vi "Is TLS.vi"(8 "error in (no error)":errorcluster, 11 "WebsocketStream in":refnum<class "WebsocketStream.lvclass">) -> (0 "error out":errorcluster, 2 "Is TLS?":bool, 3 "WebsocketStream out":refnum<class "WebsocketStream.lvclass">)   [LabVIEW 2020, in "Stream-Websocket.lvlib" / "WebsocketStream.lvclass"]
uses:
  WebsocketStream.lvclass
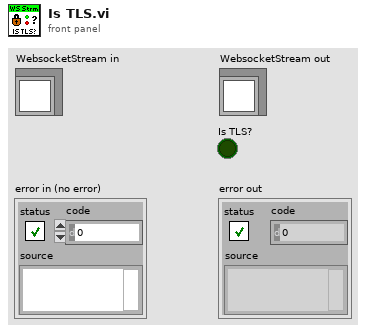
[diagram p1: front panel]
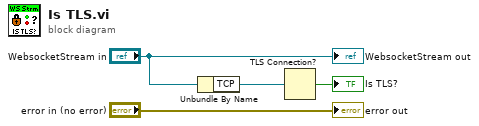
[diagram p0: block diagram]
diagram:
  n1 = Unbundle By Name("WebsocketStream in") -> ("TCP"=w2:refnum<k5>)
  n2 = TLS Connection?(1:w2) -> (0:→"Is TLS?":bool)
  "error out" <- "error in (no error)"
  "WebsocketStream out" <- "WebsocketStream in"
